vi "Parse Start Addr.vi"(8 "error in (no error)":errorcluster, 11 "Addr in":string) -> (0 "error out":errorcluster, 3 "Addr out":u16)   [LabVIEW 2018, in "Config Parser BML.lvlib" / "Config Parser BML.lvclass"]
uses:
  Config Parser BML.lvclass
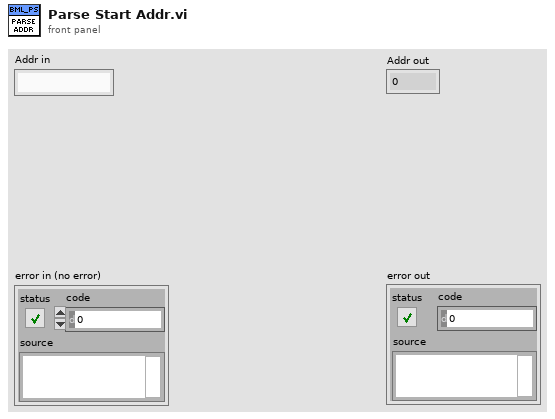
[diagram p1: front panel]
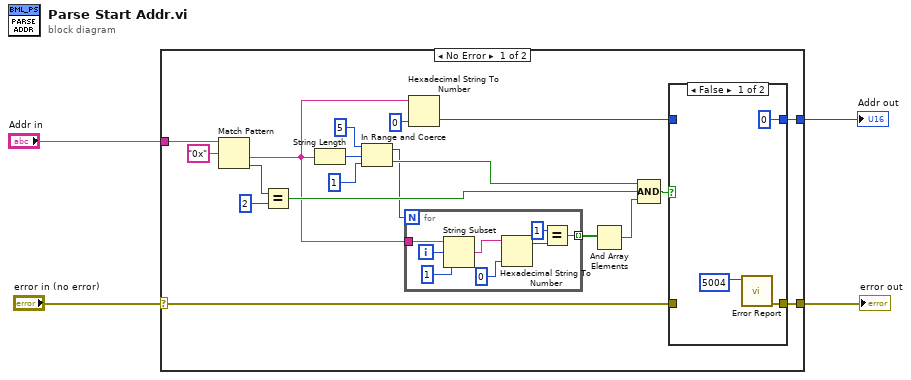
[diagram p0: block diagram]
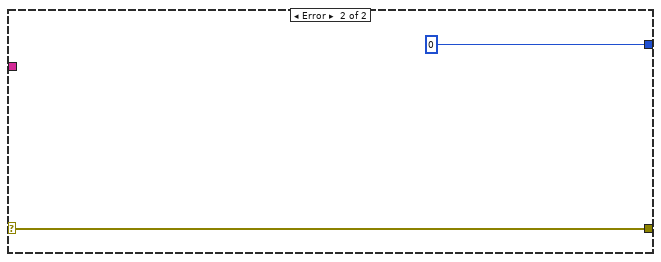
[diagram p3: hidden frame]
diagram:
  n1 = case shown="No Error" "error in (no error)" {
    selector: "error in (no error)" -> [w16 w38]
    tunnel: "Addr in" -> [w23 _]
    tunnel: [w14 w38] -> w2
    tunnel: [w13 u16 0] -> w1
    frame No Error {
      n2 = Match Pattern(string=w23, regular expression="0x") -> (after substring=w7:string, offset past match=w21:i32)  [unwired: 1 in, 2 out]
      n3 = Equal?(x=w21, y=2) -> (x = y?=w18:bool)
      n4 = String Length(string=w7) -> (length=w12:i32)
      n5 = In Range and Coerce(upper limit=5, x=w12, lower limit=1 ("upper limit")) -> (coerced(x)=w8:i32, In Range?=w9:bool)
      n6 = for {
        N: w8 -> [_]
        tunnel: w7 -> [w31]
        tunnel: [w24] -> w6 mode=indexing
        i -> [w30]
        n7 = String Subset(string=w31, offset (0)=w30, length (rest)=1 ("length (rest)")) -> (substring=w28:string)
        n8 = Hexadecimal String To Number(string=w28, default (0uL)=u16 0 ("Addr out")) -> (offset past number=w26:i32)  [unwired: 1 in, 1 out]
        n9 = Equal?(x=1, y=w26) -> (x = y?=w24:bool)
      }
      n10 = Hexadecimal String To Number(string=w7, default (0uL)=u16 0 ("Addr out")) -> (number=w15:u16)  [unwired: 1 in, 1 out]
      n11 = And Array Elements(Boolean array=w6) -> (logical AND=w5:bool)
      n12 = Compound Arithmetic op=AND(w9, w18, w5) -> (w17:bool)
      n13 = case shown="False" w17 {
        tunnel: w16 -> [_ w36]
        tunnel: w15 -> [_ w35]
        tunnel: [w33 w36] -> w14
        tunnel: [u16 0 w35] -> w13
        frame False {
          n14 = call "Error Report.vi"("Error Code"=i16 5004) -> ("error out"=w33:errorcluster)  [unwired: 10 in]
        }
        frame True {
        }
      }
    }
    frame Error {
    }
  }
  "error out" <- w2
  "Addr out" <- w1
